vi "5302GetXY.vi"(8 "error in (no error)":errorcluster, 11 "VISA Resource Name":refnum<visa-resource-name>) -> (0 "error out":errorcluster, 1 "Y":dbl, 2 "X":dbl, 3 "VISA Resource Name Out":refnum<visa-resource-name>, 4 "data string":string, 5 "Sevsitivity":dbl format="%.4e")   [LabVIEW 2015]
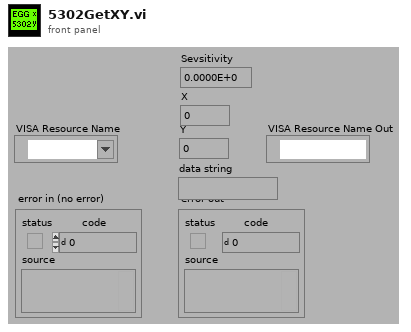
[diagram p1: front panel]
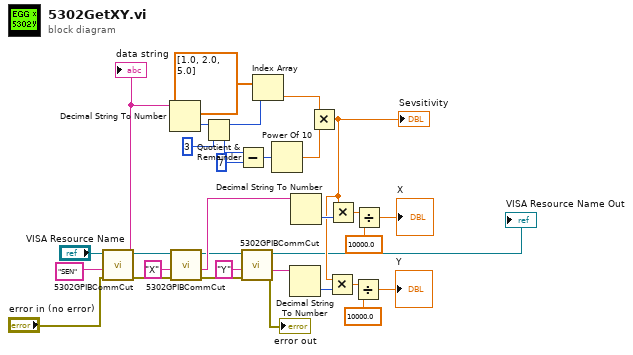
[diagram p0: block diagram]
diagram:
  n1 = call "5302GPIBCommCut.vi"("error in (no error)"="error in (no error)", "data string in"="SEN" ("data string"), "VISA Resource Name"="VISA Resource Name") -> ("error out"=w20:errorcluster, "data string out"=w28:string, "VISA Resource Name Out"=w3:refnum<visa-resource-name>)  [unwired: 2 in, 4 out]
  "data string" <- w28
  n2 = Decimal String To Number(string=w28) -> (number=w27:i32)  [unwired: 1 in, 2 out]
  n3 = call "5302GPIBCommCut.vi"("error in (no error)"=w20, "data string in"="X", "VISA Resource Name"=w3) -> ("error out"=w18:errorcluster, "data string out"=w15:string, "VISA Resource Name Out"=w2:refnum<visa-resource-name>)  [unwired: 2 in, 4 out]
  n4 = Quotient & Remainder(x=w27, y=3) -> (x-y*floor(x/y)=w23:i32, floor(x/y)=w25:i32)
  n5 = Subtract(x=w25, y=7) -> (x-y=w26:i32)
  n6 = call "5302GPIBCommCut.vi"("error in (no error)"=w18, "data string in"="Y", "VISA Resource Name"=w2) -> ("error out"=→"error out":errorcluster, "data string out"=w6:string, "VISA Resource Name Out"=→"VISA Resource Name Out":refnum<visa-resource-name>)  [unwired: 2 in, 4 out]
  n7 = Index Array(array=dbl[] [1.0, 2.0, 5.0] ("Input Array"), index=w23) -> (element=w21:dbl)
  n8 = Power Of 10(x=w26) -> (10^x=w29:dbl)
  n9 = Decimal String To Number(string=w6) -> (number=w10:i32)  [unwired: 1 in, 2 out]
  n10 = Decimal String To Number(string=w15) -> (number=w14:i32)  [unwired: 1 in, 2 out]
  n11 = Multiply(x=w21, y=w29) -> (x*y=w5:dbl)
  "Sevsitivity" <- w5
  n12 = Multiply(x=w5, y=w10) -> (x*y=w9:dbl)
  n13 = Multiply(x=w5, y=w14) -> (x*y=w13:dbl)
  n14 = Divide(x=w9, y=10000.0) -> (x/y=→"Y":dbl)
  n15 = Divide(x=w13, y=10000.0) -> (x/y=→"X":dbl)
